vi "FFT1D(CuLab).vi"() -> ()   [LabVIEW 2020]
uses:
  9db68642-0dcb-498b-b44a-62aa3c0a4411.vi
  65ef9bab-b20b-4f39-8830-9ccf3097e1d2.vi
  <vilib>/Analysis/baseanly.llb/Mean (DBL).vi
  <vilib>/Utility/High Resolution Relative Seconds.vi
  <vilib>/Ngene/CuLab - GPU Accelerated Toolkit/Toolkit/Low_Level/Tensor_Classes/T_Children/T1D/T1D_Children/T1D_CSG/Create.vi
  <vilib>/Ngene/CuLab - GPU Accelerated Toolkit/Toolkit/Low_Level/Tensor_Classes/T_Children/T1D/T1D_Children/T1D_CSG/Push.vi
  <vilib>/Ngene/CuLab - GPU Accelerated Toolkit/Toolkit/API/Signal Processing/Transforms/CU_FFT/T1D/CU_FFT_T1D_C2C.vi
  <vilib>/Ngene/CuLab - GPU Accelerated Toolkit/Toolkit/Low_Level/Tensor_Classes/T_Children/T1D/T1D_Children/T1D_CSG/Pull_to_DVR.vi
  <vilib>/Utility/file.llb/Write Delimited Spreadsheet (string).vi
  <vilib>/Analysis/NI_AALBase.lvlib
  <vilib>/Ngene/CuLab - GPU Accelerated Toolkit/Toolkit/CuLab.lvlib
  <vilib>/Ngene/CuLab - GPU Accelerated Toolkit/Toolkit/Low_Level/Tensor_Classes/T_Children/T1D/T1D_Children/T1D_CSG/T1D_CSG.lvclass
panel:
  out "error out":errorcluster
  out "Results":dbl[](graph)=[0.04420666470347593, 0.049566663801670074, 0.05085333153450241, 0.07171333224202196, 0.17785333232798925, 0.38550666746838635, 0.5215933323294545, 1.0454066708916798, 1.5011866664281115, 1.453733335559567, 2.917260000443396, 6.588726666329118, 13.42670666538955, 26.684013333093997, 55.453253333689645, 110.90791333699599, 217.96678666626877, 478.1128466682276]
  in  "Benchmark Config":cluster{"Samples":i32, "Iteration":i32}[](array[cluster])=[{"Samples"=1024, "Iteration"=20}, {"Samples"=2048, "Iteration"=20}, {"Samples"=4096, "Iteration"=20}, {"Samples"=8192, "Iteration"=20}, {"Samples"=16384, "Iteration"=20}, {"Samples"=32768, "Iteration"=20}, {"Samples"=65536, "Iteration"=20}, {"Samples"=131072, "Iteration"=20}, {"Samples"=262144, "Iteration"=20}, {"Samples"=524288, "Iteration"=20}, {"Samples"=1048576, "Iteration"=20}, {"Samples"=2097152, "Iteration"=20}, {"Samples"=4194304, "Iteration"=20}, {"Samples"=8388608, "Iteration"=20}, {"Samples"=16777216, "Iteration"=20}, {"Samples"=33554432, "Iteration"=20}, {"Samples"=67108864, "Iteration"=20}, {"Samples"=134217728, "Iteration"=20}] {"Samples" format="%#.3p"}
  out "Results(ms)":dbl[](array[numeric])=[0.04420666470347593, 0.049566663801670074, 0.05085333153450241, 0.07171333224202196, 0.17785333232798925, 0.38550666746838635, 0.5215933323294545, 1.0454066708916798, 1.5011866664281115, 1.453733335559567, 2.917260000443396, 6.588726666329118, 13.42670666538955, 26.684013333093997, 55.453253333689645, 110.90791333699599, 217.96678666626877, 478.1128466682276] format="%.8f"
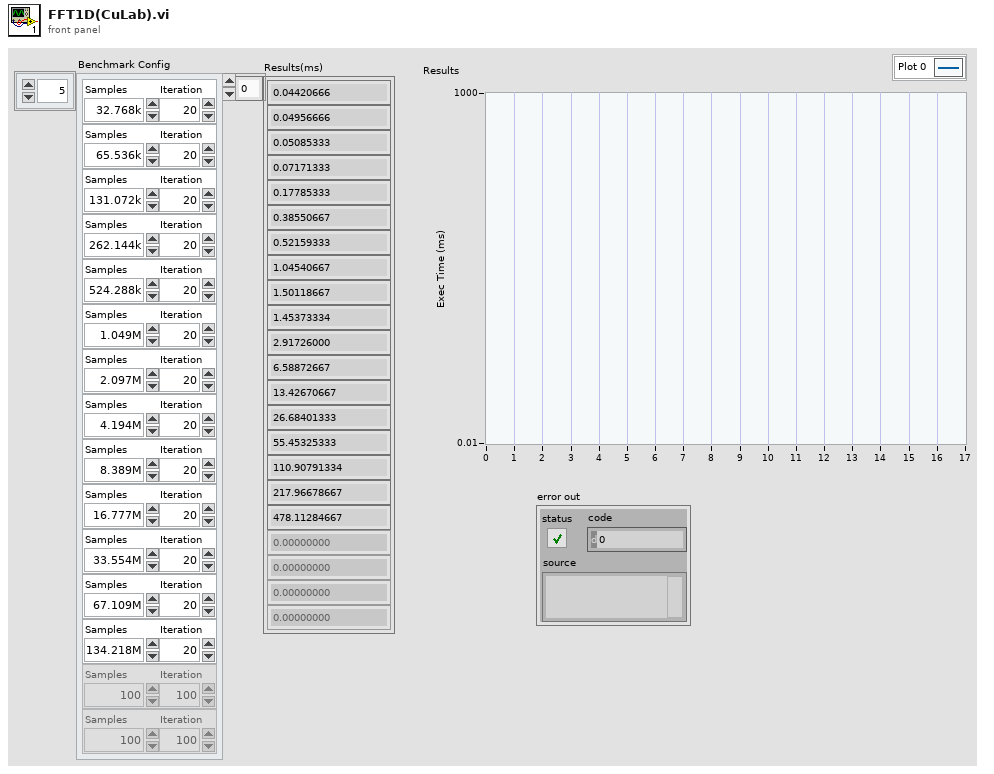
[diagram p1: front panel]
types:
  T1 = typedef "CuLab.lvlib/CuLab_Data_ref_1D_CSG.ctl" = refnum<data-value>
  T2 = typedef "CuLab.lvlib/Properties.ctl" = cluster{"Device ID":i32, "Name":string}
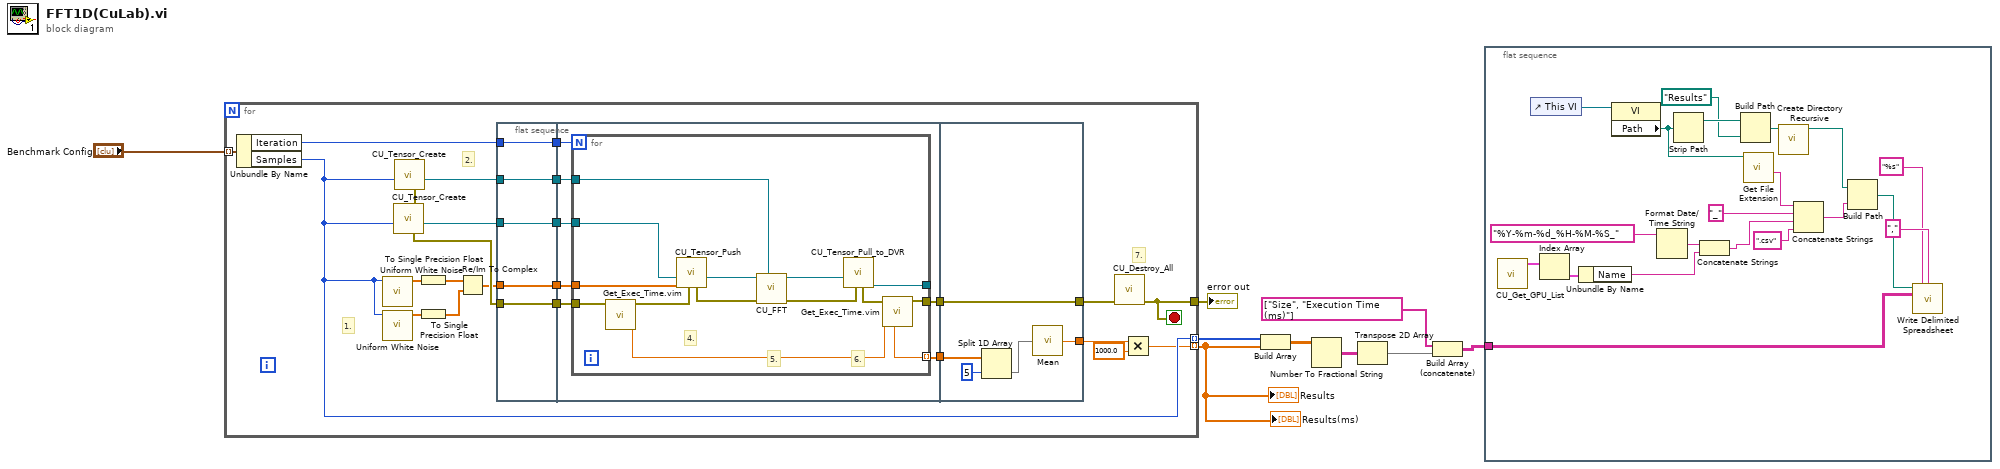
[diagram p0: block diagram]
diagram:
  n1 = for {
    tunnel: "Benchmark Config" -> [w33] mode=indexing
    tunnel: [w26] -> w1
    tunnel: [w11] -> w2 mode=indexing
    tunnel: [w13] -> w3 mode=indexing
    stop <- w26 stop-if-true
    # "7."
    # "2."
    # "1."
    n2 = Unbundle By Name(w33) -> ("Iteration"=w14:i32, "Samples"=w13:i32)
    n3 = call <vilib>:"Uniform White Noise.vi"("samples"=w13) -> ("uniform white noise"=w31:dbl[])  [unwired: 9 in, 1 out]
    n4 = call <vilib>:"Uniform White Noise.vi"("samples"=w13) -> ("uniform white noise"=w17:dbl[])  [unwired: 9 in, 1 out]
    n5 = call-poly <vilib>:"CU_Tensor_Create.vi"("Length"=w13) -> ("T1D_CSG out"=w30:refnum<class "T1D_CSG.lvclass">, "error out"=w28:errorcluster)  [unwired: 9 in]
    n6 = call-poly <vilib>:"CU_Tensor_Create.vi"("error in (no error)"=w28, "Length"=w13) -> ("T1D_CSG out"=w32:refnum<class "T1D_CSG.lvclass">, "error out"=w27:errorcluster)  [unwired: 8 in]
    n7 = To Single Precision Float(number=w31) -> (single precision float=w29:sgl[])
    n8 = To Single Precision Float(number=w17) -> (single precision float=w16:sgl[])
    n9 = Re/Im To Complex(1:w16, 2:w29) -> (0:w12:csg[])
    n10 = flat-sequence {
      tunnel: w27 -> [w34]
      tunnel: w12 -> [w35]
      tunnel: w14 -> [w36]
      tunnel: w30 -> [w37]
      tunnel: w32 -> [w38]
      tunnel: [w38] -> w23
      tunnel: [w37] -> w22
      tunnel: [w36] -> w21
      tunnel: [w35] -> w20
      tunnel: [w34] -> w19
      tunnel: [w41] -> w24
      tunnel: w23 -> [w45]
      tunnel: w22 -> [w44]
      tunnel: w21 -> [w40]
      tunnel: w20 -> [w43]
      tunnel: w19 -> [w42]
      tunnel: [w39] -> w15
      tunnel: [w64] -> w25
      tunnel: w24 -> [w64]
      tunnel: [w60] -> w18
      tunnel: w15 -> [w63]
      frame #0 {
      }
      frame #1 {
        n11 = for {
          N: w40 -> [_]
          tunnel: w43 -> [w47]
          tunnel: w45 -> [w55]
          tunnel: w44 -> [w57]
          tunnel: w42 -> [w49]
          tunnel: [w50] -> w41
          tunnel: [w52] -> w39 mode=indexing
          tunnel: [w46] -> _
          # "6."
          # "5."
          # "4."
          n12 = call "Get_Exec_Time.vim"("error in (no error)"=w49) -> ("T(n)"=w53:dbl, "error out"=w48:errorcluster)  [unwired: 6 in, 1 out]
          n13 = call-poly <vilib>:"CU_Tensor_Push.vi"("error in (no error)"=w48, "CPU_Data_1D_CSG"=w47, "T1D_CSG in"=w55) -> ("T1D_CSG out"=w59:refnum<class "T1D_CSG.lvclass">, "error out"=w58:errorcluster)  [unwired: 7 in]
          n14 = call-poly <vilib>:"CU_FFT.vi"("FFT {X} dest"=w57, "error in"=w58, "X"=w59) -> ("error out"=w56:errorcluster, "FFT {X}"=w54:refnum<class "T1D_CSG.lvclass">)  [unwired: 7 in]
          n15 = call-poly <vilib>:"CU_Tensor_Pull_to_DVR.vi"("error in (no error)"=w56, "T1D_CSG in"=w54) -> ("Dest out"=w46:T1, "error out"=w51:errorcluster)  [unwired: 7 in, 1 out]
          n16 = call "Get_Exec_Time.vim"("T(n-1)"=w53, "error in (no error)"=w51) -> ("error out"=w50:errorcluster, "dT"=w52:dbl)  [unwired: 5 in, 1 out]
        }
      }
      frame #2 {
        n17 = Split 1D Array(array=w63, index=5) -> (second subarray=w61:dbl[])  [unwired: 1 out]
        n18 = call-poly <vilib>:"Mean.vi"("X"=w61) -> ("mean"=w60:dbl)  [unwired: 1 out]
      }
    }
    n19 = call <vilib>:"CU_Destroy_All.vi"("error in"=w25) -> ("error out"=w26:errorcluster)  [unwired: 10 in]
    n20 = Multiply(x=w18, y=1000.0) -> (x*y=w11:dbl)
  }
  "Results(ms)" <- w2
  "Results" <- w2
  "error out" <- w1
  n21 = Build Array(w3, w2) -> (w9:dbl[][])
  n22 = Number To Fractional String(number=w9) -> (F-format string=w8:string[][])  [unwired: 3 in]
  n23 = Transpose 2D Array(2D array=w8) -> (transposed array=w7:string[][])
  n24 = Build Array (concatenate)(string[] ["Size", "Execution Time (ms)"] ("element"), w7) -> (w5:string[][])
  n25 = flat-sequence {
    tunnel: w5 -> [w84]
    frame #0 {
      n26 = call <vilib>:"CU_Get_GPU_List.vi"() -> ("Devices"=w68:T2[])  [unwired: 10 in, 1 out]
      n27 = control-ref of="This VI"() -> (w78:refnum<vi>)
      n28 = Index Array(array=w68) -> (element=w67:T2)  [unwired: 1 in]
      n29 = Unbundle By Name(w67) -> ("Name"=w66:string)
      n30 = property class="VI"(reference=w78) -> ("Path"=w73:path)  [unwired: 1 in, 2 out]
      n31 = Format Date/Time String(time format string (%c)="%Y-%m-%d_%H-%M-%S_") -> (date/time string=w69:string)  [unwired: 2 in]
      n32 = Strip Path(path=w73) -> (stripped path=w77:path)  [unwired: 1 out]
      n33 = Concatenate Strings(w69, w66) -> (w65:string)
      n34 = Build Path(base path=w77, name or relative path=path "Results") -> (appended path=w76:path)
      n35 = call <vilib>:"Get File Extension.vi"("file"=w73) -> ("filename without extension"=w72:string)  [unwired: 6 in, 4 out]
      n36 = call <vilib>:"Create Directory Recursive.vi"("directory"=w76) -> ("directory copy"=w74:path)  [unwired: 4 in, 2 out]
      n37 = Concatenate Strings(w72, "_" ("string"), w65, ".csv" ("string")) -> (w82:string)
      n38 = Build Path(base path=w74, name or relative path=w82) -> (appended path=w83:path)
      n39 = call-poly <vilib>:"Write Delimited Spreadsheet.vi"("file path (dialog if empty)"=w83, "format (%s)"="%s", "2D data"=w84, "delimiter (\\t)"="," ("delimiter (\\t)")) -> ()  [unwired: 10 in, 2 out]
    }
  }
